vi "aal_cascaded moving average (complex input) (No State).vi"(7 "aal_cascaded moving average (complex input) state in":T1, 8 "Reset":bool, 9 "Stages":i32, 10 "N":i32=1, 11 "x":cdb[](array[numeric]) format="%_6g") -> (3 "y":cdb[](array[numeric]) format="%_6g", 5 "aal_cascaded moving average (complex input) state out":T1)   [LabVIEW 2014, in "NI_AALPro.lvlib"]
uses:
  NI_AALPro.lvlib
  lvanlys.dll
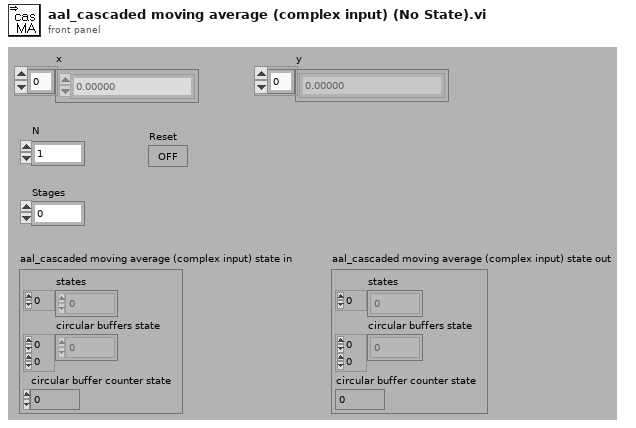
[diagram p1: front panel]
types:
  T1 = cluster{"states":cdb[], "circular buffers state":cdb[][], "circular buffer counter state":i32}
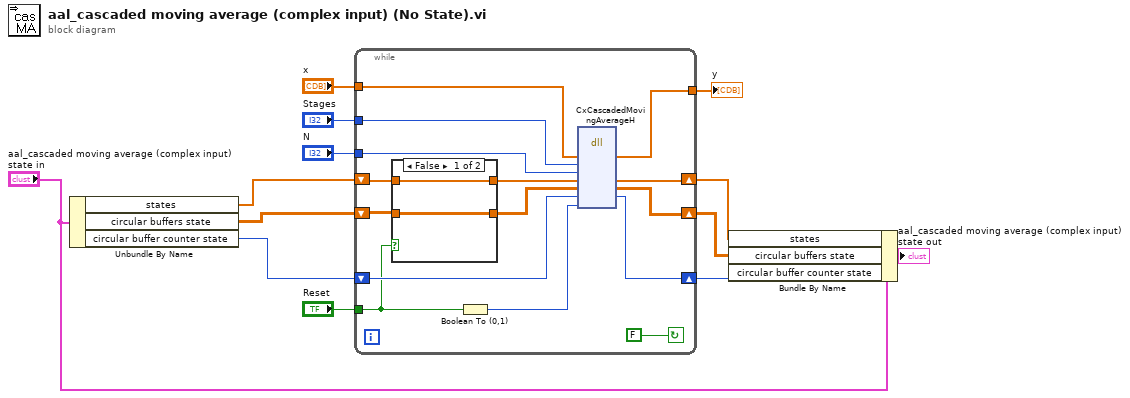
[diagram p0: block diagram]
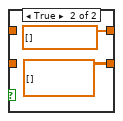
[diagram p2: hidden frame]
diagram:
  n1 = Unbundle By Name("aal_cascaded moving average (complex input) state in") -> ("states"=w7:cdb[], "circular buffers state"=w6:cdb[][], "circular buffer counter state"=w5:i32)
  n2 = while {
    tunnel: [w15] -> w10
    tunnel: "x" -> [w16]
    tunnel: "Reset" -> [w20]
    tunnel: "Stages" -> [w25]
    tunnel: "N" -> [w26]
    shift-left: w6 -> [w14]
    shift-right: [w22] -> w3
    shift-left: w5 -> [w27]
    shift-right: [w28] -> w2
    shift-left: w7 -> [w18]
    shift-right: [w17] -> w4
    stop <- FALSE continue-if-true
    n3 = case shown="False" w20 {
      tunnel: [w30 cdb[][] [] ("Array Constant")] -> w21
      tunnel: w14 -> [w30 _]
      tunnel: [w29 cdb[] [] ("Array Constant")] -> w19
      tunnel: w18 -> [w29 _]
      frame False {
      }
      frame True {
      }
    }
    n4 = Boolean To (0,1)(Boolean=w20) -> (0, 1=w24:i16)
    n5 = dll-call lib="C:/Program Files (x86)/National Instruments/LabVIEW 2014/resource/lvanlys.*" fn="CxCascadedMovingAverageH"("xH"=w16, "stages"=w25, "N"=w26, "states"=w19, "ibuf"=w21, "ibuf_cnt"=w27, "Reset"=w24) -> ("xH"=w15:cdb[], "states"=w17:cdb[], "ibuf"=w22:cdb[][], "ibuf_cnt"=w28:i32)  [unwired: 7 in, 2 out]
  }
  "y" <- w10
  n6 = Bundle By Name(cluster="aal_cascaded moving average (complex input) state in", "states"=w4, "circular buffers state"=w3, "circular buffer counter state"=w2) -> (→"aal_cascaded moving average (complex input) state out":T1)
